vi "MIF_N_num_cont-de-obs.vi"(8 "ni-OBS":u32[](array[numeric]), 9 "X-OBS":dbl[](array[numeric]), 11 "Xi-classes":dbl[](array[numeric])) -> (2 "N-MIF":u32[](array[numeric]))   [LabVIEW 2010, in "lv_02.lvlib"]
doc: "A partir des observations :\n- MIF : Classes - > X-obs est le tableau xic et le tableau des effectifs ni-OBS\n- NON MIF : X-obs contient les valeurs observées xi\nOn retourne le tableau ni associé à chaque classe dont les limites sont données par le tableau xi-MIF"
uses:
  lv_02.lvlib
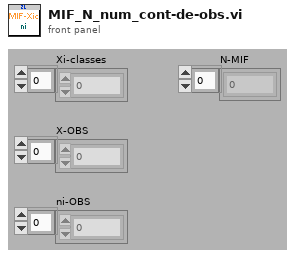
[diagram p1: front panel]
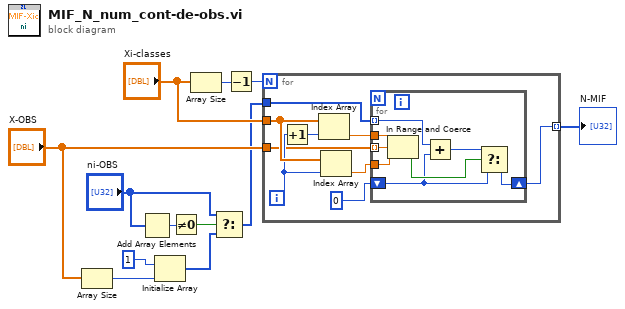
[diagram p0: block diagram]
diagram:
  n1 = Array Size(array="X-OBS") -> (size(s)=w3:i32)
  n2 = Add Array Elements(numeric array="ni-OBS") -> (sum=w8:u32)
  n3 = Initialize Array(1 ("x_deb"), w3) -> (w2:i32[])
  n4 = Not Equal To 0?(x=w8) -> (x != 0?=w7:bool)
  n5 = Array Size(array="Xi-classes") -> (size(s)=w12:i32)
  n6 = Select(t="ni-OBS", s=w7, f=w2) -> (s? t:f=w1:u32[])
  n7 = Decrement(x=w12) -> (x-1=w11:i32)
  n8 = for {
    N: w11 -> [_]
    tunnel: "Xi-classes" -> [w20]
    tunnel: "X-OBS" -> [w18]
    tunnel: w1 -> [w14]
    tunnel: [w13] -> w9 mode=indexing
    i -> [w19]
    n9 = Increment(x=w19) -> (x+1=w21:i32)
    n10 = Index Array(array=w20, index=w21) -> (element=w17:dbl)
    n11 = Index Array(array=w20, index=w19) -> (element=w16:dbl)
    n12 = for {
      tunnel: w18 -> [w25] mode=indexing
      tunnel: w17 -> [w29]
      tunnel: w16 -> [w28]
      shift-right: [w27] -> w13
      shift-left: 0 -> [w22]
      tunnel: w14 -> [w24] mode=indexing
      n13 = In Range and Coerce(upper limit=w29, x=w25, lower limit=w28) -> (In Range?=w26:bool)  [unwired: 1 out]
      n14 = Add(x=w24, y=w22) -> (x+y=w23:u32)
      n15 = Select(t=w23, s=w26, f=w22) -> (s? t:f=w27:u32)
    }
  }
  "N-MIF" <- w9
